vi "zapis.vi"(4 "Wybranie tabeli z bazy danych":string, 5 "Wciœniêcie powoduje wykonanie akcji":bool, 6 "Wybranie bazy danych - plik .UDL":path, 7 "Zapis / Odczyt":string(combo)="Zapis", 8 "PM10":dbl, 9 "PM25":dbl, 10 "PM1":dbl, 11 "TIME":dbl) -> (3 "DANE WYJŒCIOWE":dbl[][](array[numeric]))   [LabVIEW 2019]
uses:
  <vilib>/addons/database/Connection.llb/DB Tools Open Connec (Path).vi
  <vilib>/addons/database/_DB Variant To Data/Database Variant To Data.xnode
  <vilib>/addons/database/NI_Database_API.lvlib
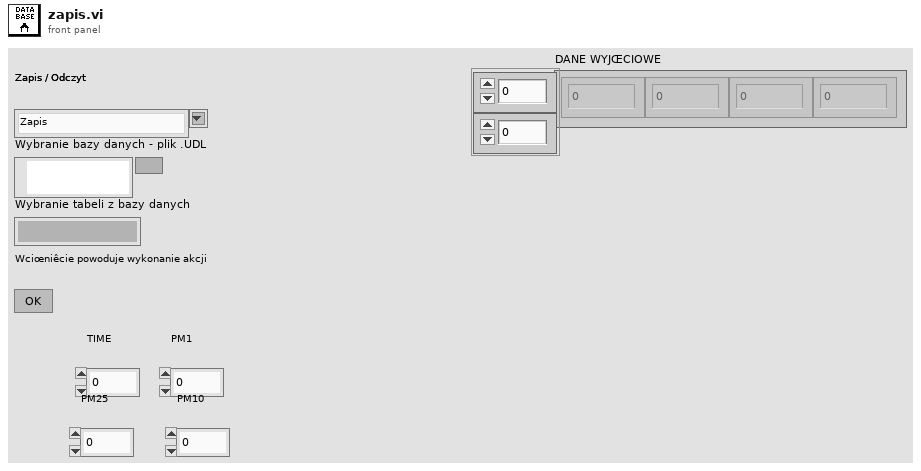
[diagram p1: front panel]
types:
  T1 = cluster{"TIME":dbl, "PM1":dbl, "PM25":dbl, "PM10":dbl}
  T2 = typedef "NI_Database_API.lvlib/Conn ObjectReference.ctl" = refnum<k1>
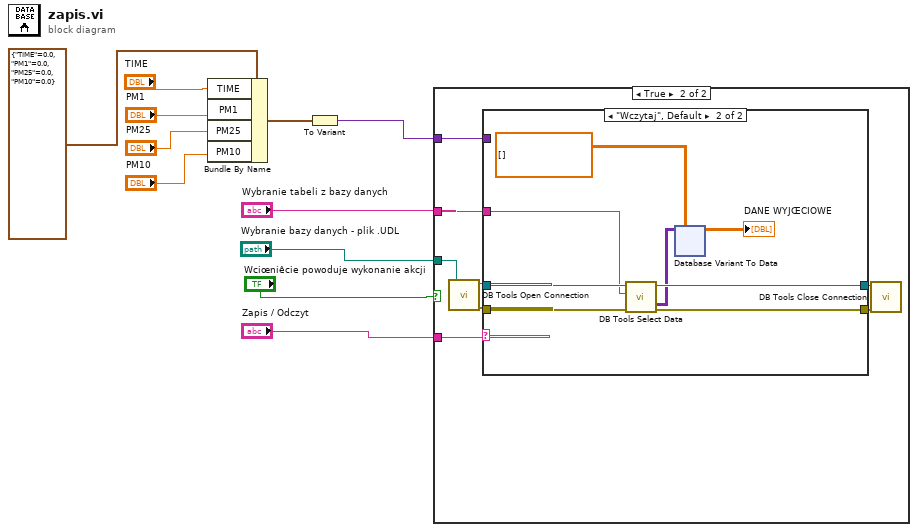
[diagram p0: block diagram]
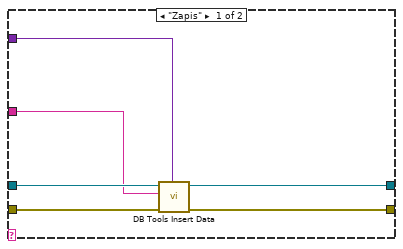
[diagram p3: hidden frame]
diagram:
  n1 = Bundle By Name(cluster=T1 {"TIME"=0.0, "PM1"=0.0, "PM25"=0.0, "PM10"=0.0}, "TIME"="TIME", "PM1"="PM1", "PM25"="PM25", "PM10"="PM10") -> (w2:T1)
  n2 = To Variant(anything=w2) -> (Variant=w1:variant)
  n3 = case shown="True" "Wciœniêcie powoduje wykonanie akcji" {
    tunnel: "Zapis / Odczyt" -> [_ w19]
    tunnel: "Wybranie bazy danych - plik .UDL" -> [_ w18]
    tunnel: "Wybranie tabeli z bazy danych" -> [_ w13]
    tunnel: w1 -> [_ w12]
    frame False {
    }
    frame True {
      n4 = call-poly <vilib>:"DB Tools Open Connection.vi"("connection information"=w18) -> ("error out"=w17:errorcluster, "connection reference"=w16:T2)  [unwired: 7 in]
      n5 = case shown="\"Wczytaj\", Default" w19 {
        tunnel: [w22 w33] -> w15
        tunnel: [w23 w32] -> w14
        tunnel: w17 -> [w24 w31]
        tunnel: w16 -> [w25 w30]
        tunnel: w13 -> [w21 w27]
        tunnel: w12 -> [w20 _]
        frame "Zapis" {
          n6 = call <vilib>:"DB Tools Insert Data.vi"("data"=w20, "error in (no error)"=w24, "table"=w21, "connection reference"=w25) -> ("error out"=w22:errorcluster, "connection reference out"=w23:T2)  [unwired: 6 in]
        }
        frame "Wczytaj", Default {
          n7 = call <vilib>:"DB Tools Select Data.vi"("error in (no error)"=w31, "table"=w27, "connection reference"=w30) -> ("error out"=w33:errorcluster, "data"=w29:variant[][], "connection reference out"=w32:T2)  [unwired: 3 in]
          n8 = xnode "Database Variant To Data"("database variant"=w29, "type"=dbl[][] []) -> ("data"=→"DANE WYJŒCIOWE":dbl[][])  [unwired: 1 in, 1 out]
        }
      }
      n9 = call <vilib>:"DB Tools Close Connection.vi"("error in (no error)"=w15, "connection reference"=w14) -> ()  [unwired: 5 in, 1 out]
    }
  }
